vi "read-cluster-io-name.vi"(8 "error in (no error)":errorcluster, 11 "dbc in":refnum<class "dbc.lvclass">) -> (0 "error out":errorcluster, 2 "XNET Cluster":refnum<k21>, 3 "dbc out":refnum<class "dbc.lvclass">)   [LabVIEW 2015, in "dbc.lvclass"]
uses:
  dbc.lvclass
  <vilib>/xnet/xnet.llb/XNET String To IO Name (Cluster).vi
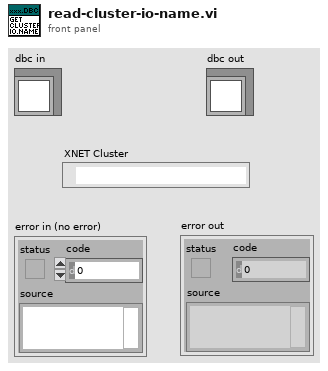
[diagram p1: front panel]
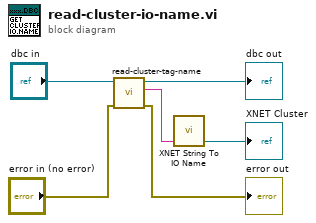
[diagram p0: block diagram]
diagram:
  n1 = call "read-cluster-tag-name.vi"("error in (no error)"="error in (no error)", "dbc in"="dbc in") -> ("error out"=→"error out":errorcluster, "tag.cluster"=w4:string, "dbc out"=→"dbc out":refnum<class "dbc.lvclass">)  [unwired: 7 in]
  n2 = call-poly <vilib>:"XNET String To IO Name.vi"("string"=w4) -> ("XNET Cluster"=→"XNET Cluster":refnum<k21>)  [unwired: 4 out]
